vi "AD7747 READ 16 DUT.vi"(8 "error in":errorcluster) -> (0 "error out":errorcluster, 3 "AD7747 Values":string[][](table))   [LabVIEW 2012]
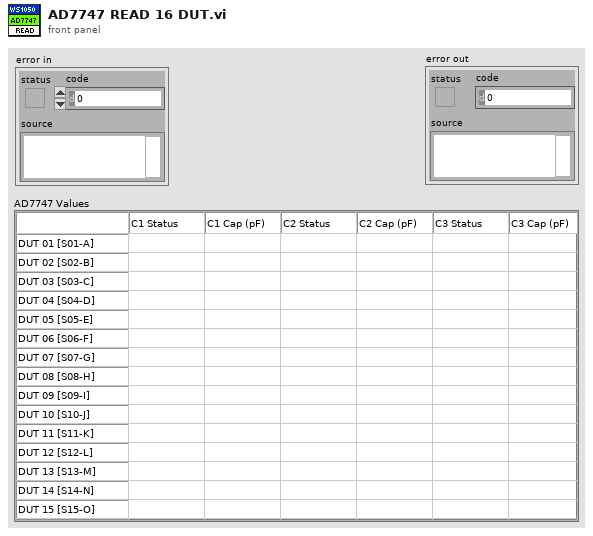
[diagram p1: front panel]
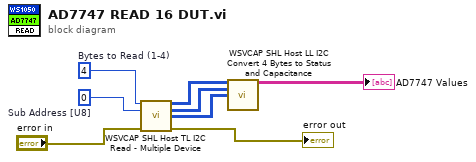
[diagram p0: block diagram]
diagram:
  w7 = u8 4  # Bytes to Read (1-4)
  w8 = u8 0  # Sub Address [U8]
  n1 = call "WSVCAP SHL Host TL I2C Read - Multiple Device.vi"("Bytes to Read (1-4)"=w7, "Sub Address [U8]"=w8, "error in"="error in") -> ("C1:1-16 Read Data [U8]"=w6:u8[][], "C2:1-16 Read Data [U8]"=w5:u8[][], "C3:1-16 Read Data [U8]"=w3:u8[][], "error out"=→"error out":errorcluster)  [unwired: 9 in]
  n2 = call "WSVCAP SHL Host LL I2C Convert 4 Bytes to Status and Capacitance.vi"("C1:1-16 Read Data [U8]"=w6, "C2_1-16 Read Data [U8]"=w5, "C3_1-16 Read Data [U8]"=w3) -> ("AD7747 Values"=→"AD7747 Values":string[][])  [unwired: 12 in]
